vi "Launch Monitor-Pulse.vi"() -> ()   [LabVIEW 2016]
uses:
  Monitor-Pulse/Monitor-Pulse.lvclass
  D:/github/Measure_core/Controllers/Application Controller/Application Controller.lvclass
  Measure_core/Controllers/Application Controller/Load App.vi
  Measure_core/Controllers/Application Controller/Application Controller.lvclass
panel:
  out "Waiting Lights":T1
  out "Current action:":string
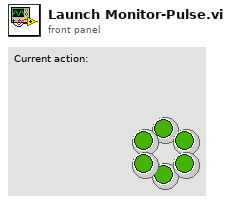
[diagram p1: front panel]
types:
  T1 = cluster{"DNL_wait 1":bool, "DNL_wait 1":bool, "DNL_wait 1":bool, "DNL_wait 1":bool, "DNL_wait 1":bool, "DNL_wait 1":bool}
  T2 = cluster{"[0]":bool, "[1]":bool, "[2]":bool, "[3]":bool, "[4]":bool, "[5]":bool}
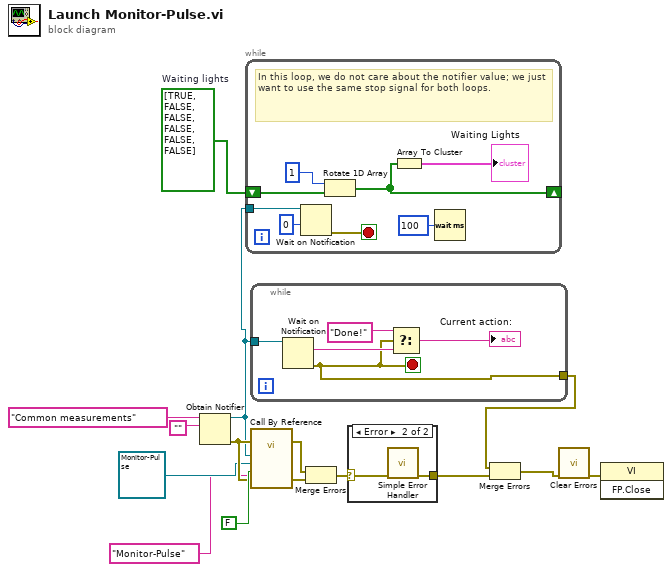
[diagram p0: block diagram]
diagram:
  w4 = bool[] [TRUE, FALSE, FALSE, FALSE, FALSE, FALSE]  # Waiting lights
  n1 = Obtain Notifier(name (unnamed)="Common measurements", notification data type="") -> (notifier out=w3:refnum<notifier>, error out=w10:errorcluster)  [unwired: 2 in, 1 out]
  n2 = while {
    shift-right: [w17] -> _
    shift-left: w4 -> [w19]
    tunnel: w3 -> [w21]
    stop <- w23 stop-if-true
    # "In this loop, we do not care about the notifier value; we just want to use the same stop signal for both loops."
    n3 = Wait on Notification(notifier=w21, timeout in ms (-1)=0) -> (error out=w23:errorcluster)  [unwired: 2 in, 3 out]
    n4 = Rotate 1D Array(1:w19, 2:1 ("n")) -> (0:w17:bool[])
    n5 = Array To Cluster(array=w17) -> (cluster=→"Waiting Lights":T2)
    n6 = Wait (ms)(milliseconds to wait=u32 100) -> ()  [unwired: 1 out]
  }
  n7 = while {
    tunnel: w3 -> [w28]
    tunnel: [w24] -> w5
    stop <- w24 stop-if-true
    n8 = Wait on Notification(notifier=w28) -> (notification=w26:string, error out=w24:errorcluster)  [unwired: 3 in, 2 out]
    n9 = Select(t="Done!" ("notification"), s=w24, f=w26) -> (s? t:f=→"Current action:":string)
  }
  n10 = call-by-ref "?"(error in=w10, "Name"="Monitor-Pulse", "Error In"=w10, "Open Actor Core front panel? (F)"=FALSE, "Application Controller.lvclass"=refnum<class "Monitor-Pulse.lvclass"> refnum ("Monitor-Pulse.lvclass"), "Status Notifier"=w3) -> (error out=w13:errorcluster, "Error Out"=w9:errorcluster)  [unwired: 7 in, 1 out]
  n11 = Merge Errors(w13, w9) -> (w14:errorcluster)
  n12 = case shown="Error" w14 {
    selector: w14 -> [w29 w31]
    tunnel: [w29 w30] -> w7
    frame No Error {
    }
    frame Error {
      n13 = call <vilib>:"Simple Error Handler.vi"("error in (no error)"=w31) -> ("error out"=w30:errorcluster)  [unwired: 4 in, 4 out]
    }
  }
  n14 = Merge Errors(w5, w7) -> (w6:errorcluster)
  n15 = call <vilib>:"Clear Errors.vi"("error in (no error)"=w6) -> ("error out"=w15:errorcluster)  [unwired: 5 in, 1 out]
  n16 = invoke class="VI" method="FP.Close"(error in=w15) -> ()  [unwired: 2 in, 3 out]
